vi "Write Monitor File.vi"(8 "error in (no error)":errorcluster, 9 "Open plot":bool, 10 "Monitor File":path, 11 "Monitor-Pulse in":refnum<class "Application Controller.lvclass">) -> (0 "error out":errorcluster, 3 "Monitor-Pulse out":refnum<class "Application Controller.lvclass">)   [LabVIEW 2019, in "Application Controller.lvclass"]
uses:
  Application Controller.lvclass
  Plots/Plot types.ctl
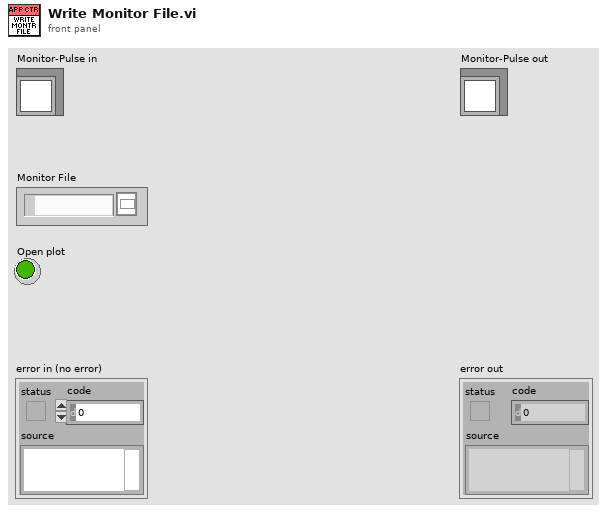
[diagram p1: front panel]
types:
  T1 = typedef "Plot types.ctl" = enum16{"Waveform Plot", "XY Plot", "Full XY"}
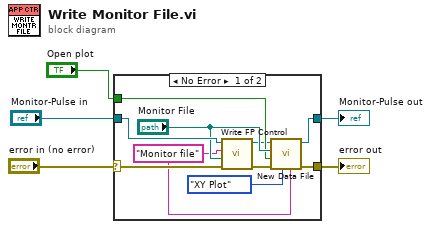
[diagram p0: block diagram]
diagram:
  n1 = case shown="No Error" "error in (no error)" {
    selector: "error in (no error)" -> [w14 w17]
    tunnel: [w7 w17] -> w4
    tunnel: [w9 w16] -> w2
    tunnel: "Monitor-Pulse in" -> [w15 w16]
    tunnel: "Open plot" -> [w11 _]
    frame No Error {
      w6 = "Monitor file" ("Control Name")
      n2 = call-dynamic "Write FP Control.vi"("error in (no error)"=w14, "Control Value"="Monitor File", "Control Name"=w6, "Measure Object in"=w15) -> ("error out"=w8:errorcluster, "Measure Object out"=w10:refnum<class "Application Controller.lvclass">)  [unwired: 6 in]
      n3 = call-dynamic "New Data File.vi"("Plot group"=w6, "Plot type"=Plot_types."XY Plot", "error in (no error)"=w8, "New plot if not open"=w11, "File"="Monitor File", "Application Controller in"=w10) -> ("error out"=w7:errorcluster, "Application Controller out"=w9:refnum<class "Application Controller.lvclass">)  [unwired: 4 in]
    }
    frame Error {
    }
  }
  "error out" <- w4
  "Monitor-Pulse out" <- w2
